vi "KEY_PRESS.vi"(0 "device ID":refnum<k1>, 1 "error in (no error)":errorcluster) -> (2 "device ID 2":refnum<k1>, 3 "Direction 2":T1, 4 "error out":errorcluster)   [LabVIEW 2015]
uses:
  DIR GAME.ctl
  <vilib>/Utility/inputDevices.llb/keyboardAcquire.vi
panel:
  out "keys pressed 2":T2(array[ring])
  out "keys pressed":T2(array[ring])
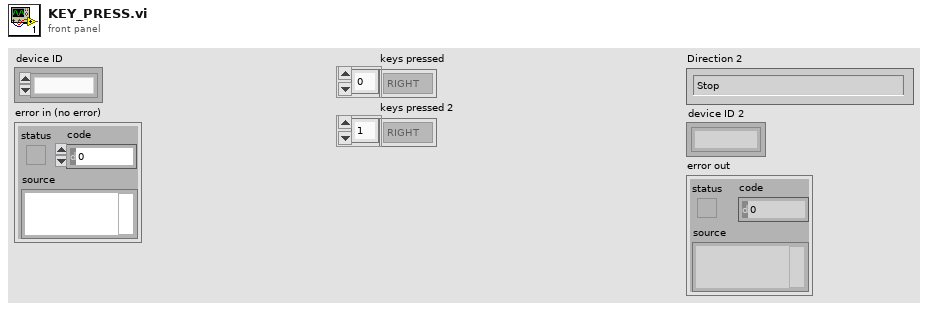
[diagram p1: front panel]
types:
  T1 = typedef "DIR GAME.ctl" = enum16{"Stop", "Front", "FR", "Right", "BR", "Back", "BL", "Left", "FL"}
  T2 = enum16{"0", "1", "2", "3", "4", "5", "6", "7", "8", "9", "A", "B", "C", "D", "E", "F", "G", "H", "I", "J", "K", "L", "M", "N", "O", "P", "Q", "R", "S", "T", "U", "V", "W", "X", "Y", "Z", "F1", "F2", "F3", "F4", "F5", "F6", "F7", "F8", "F9", "F10", "F11", "F12", "F13", "F14", "F15", "ADD", "BACK", "BACKSLASH", "CAPITAL", "COMMA", "DECIMAL", "DELETE", "DIVIDE", "DOWN", "END", "EQUALS", "ESCAPE", "GRAVE (`)", "HOME", "INSERT", "LBRACKET", "LCONTROL", "LEFT", "L ALT", "LSHIFT", "LWIN", "MINUS", "MULTIPLY", "NEXT", "NUMLOCK", "NUMPAD_0", "NUMPAD_1", "NUMPAD_2", "NUMPAD_3", "NUMPAD_4", "NUMPAD_5", "NUMPAD_6", "NUMPAD_7", "NUMPAD_8", "NUMPAD_9", "PAUSE", "PERIOD", "PRIOR (PG UP)", "RBRACKET", "RCONTROL", "RETURN", "RIGHT", "R ALT", "RSHIFT", "RWIN", "SCROLL", "SEMICOLON", "SLASH", "SPACE", "SUBTRACT", "TAB", "UP", "ENTER (num pad)", "' (quote)"}[]
  T3 = enum16{"0", "1", "2", "3", "4", "5", "6", "7", "8", "9", "A", "B", "C", "D", "E", "F", "G", "H", "I", "J", "K", "L", "M", "N", "O", "P", "Q", "R", "S", "T", "U", "V", "W", "X", "Y", "Z", "F1", "F2", "F3", "F4", "F5", "F6", "F7", "F8", "F9", "F10", "F11", "F12", "F13", "F14", "F15", "ADD", "BACK", "BACKSLASH", "CAPITAL", "COMMA", "DECIMAL", "DELETE", "DIVIDE", "DOWN", "END", "EQUALS", "ESCAPE", "GRAVE (`)", "HOME", "INSERT", "LBRACKET", "LCONTROL", "LEFT", "L ALT", "LSHIFT", "LWIN", "MINUS", "MULTIPLY", "NEXT", "NUMLOCK", "NUMPAD_0", "NUMPAD_1", "NUMPAD_2", "NUMPAD_3", "NUMPAD_4", "NUMPAD_5", "NUMPAD_6", "NUMPAD_7", "NUMPAD_8", "NUMPAD_9", "PAUSE", "PERIOD", "PRIOR (PG UP)", "RBRACKET", "RCONTROL", "RETURN", "RIGHT", "R ALT", "RSHIFT", "RWIN", "SCROLL", "SEMICOLON", "SLASH", "SPACE", "SUBTRACT", "TAB", "UP", "ENTER (num pad)", "' (quote)"}
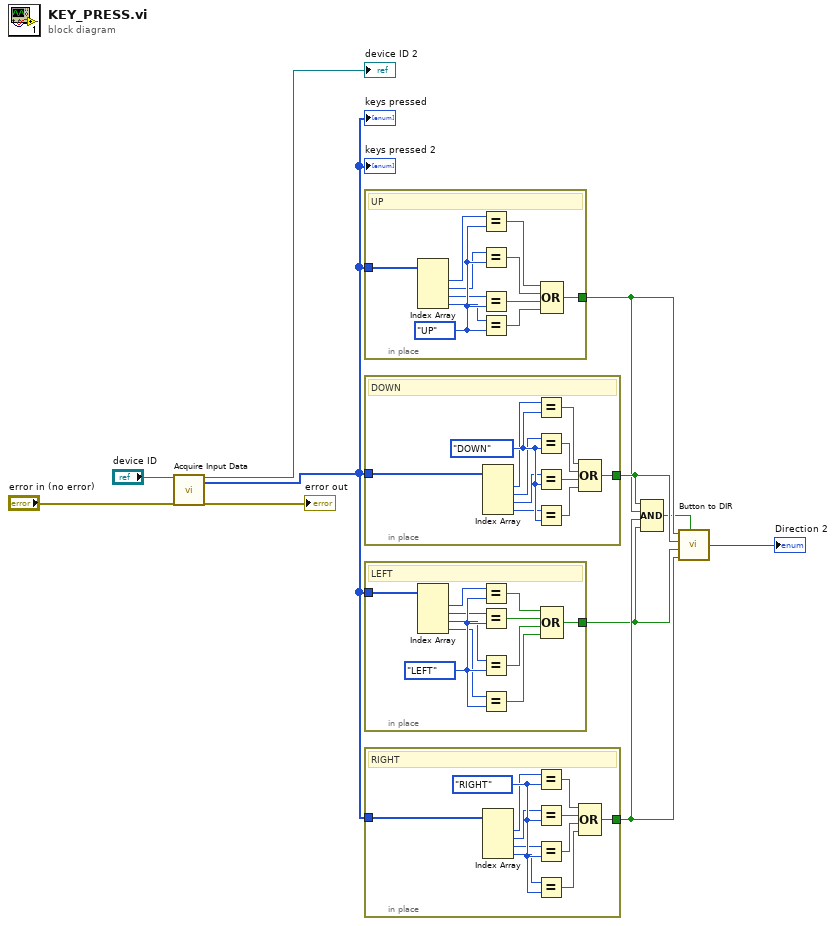
[diagram p0: block diagram]
diagram:
  n1 = call-poly <vilib>:"Acquire Input Data.vi"("device ID"="device ID", "error in (no error)"="error in (no error)") -> ("device ID"=→"device ID 2":refnum<k1>, "keys pressed"=w5:T2, "error out"=→"error out":errorcluster)  [unwired: 15 in]
  "keys pressed" <- w5
  "keys pressed 2" <- w5
  n2 = in-place {
    in-place-border: w5 -> [w13]
    in-place-border: [w12] -> w7
    w18 = T3."UP" ("element")
    # "UP"
    n3 = Index Array(array=w13) -> (element #1=w17:T3, element #2=w16:T3, element #3=w15:T3, element #4=w14:T3)  [unwired: 4 in]
    n4 = Equal?(x=w17, y=w18) -> (x = y?=w22:bool)
    n5 = Equal?(x=w16, y=w18) -> (x = y?=w21:bool)
    n6 = Equal?(x=w15, y=w18) -> (x = y?=w20:bool)
    n7 = Equal?(x=w14, y=w18) -> (x = y?=w19:bool)
    n8 = Compound Arithmetic op=OR(w22, w21, w20, w19) -> (w12:bool)
  }
  n9 = in-place {
    in-place-border: w5 -> [w24]
    in-place-border: [w23] -> w8
    w29 = T3."DOWN" ("element")
    # "DOWN"
    n10 = Index Array(array=w24) -> (element #1=w28:T3, element #2=w27:T3, element #3=w26:T3, element #4=w25:T3)  [unwired: 4 in]
    n11 = Equal?(x=w28, y=w29) -> (x = y?=w33:bool)
    n12 = Equal?(x=w27, y=w29) -> (x = y?=w32:bool)
    n13 = Equal?(x=w26, y=w29) -> (x = y?=w31:bool)
    n14 = Equal?(x=w25, y=w29) -> (x = y?=w30:bool)
    n15 = Compound Arithmetic op=OR(w33, w32, w31, w30) -> (w23:bool)
  }
  n16 = in-place {
    in-place-border: w5 -> [w35]
    in-place-border: [w34] -> w9
    w40 = T3."LEFT" ("element")
    # "LEFT"
    n17 = Index Array(array=w35) -> (element #1=w39:T3, element #2=w38:T3, element #3=w37:T3, element #4=w36:T3)  [unwired: 4 in]
    n18 = Equal?(x=w39, y=w40) -> (x = y?=w44:bool)
    n19 = Equal?(x=w38, y=w40) -> (x = y?=w43:bool)
    n20 = Equal?(x=w37, y=w40) -> (x = y?=w42:bool)
    n21 = Equal?(x=w36, y=w40) -> (x = y?=w41:bool)
    n22 = Compound Arithmetic op=OR(w44, w43, w42, w41) -> (w34:bool)
  }
  n23 = in-place {
    in-place-border: w5 -> [w46]
    in-place-border: [w45] -> w10
    w51 = T3."RIGHT" ("element")
    # "RIGHT"
    n24 = Index Array(array=w46) -> (element #1=w50:T3, element #2=w49:T3, element #3=w48:T3, element #4=w47:T3)  [unwired: 4 in]
    n25 = Equal?(x=w50, y=w51) -> (x = y?=w55:bool)
    n26 = Equal?(x=w49, y=w51) -> (x = y?=w54:bool)
    n27 = Equal?(x=w48, y=w51) -> (x = y?=w53:bool)
    n28 = Equal?(x=w47, y=w51) -> (x = y?=w52:bool)
    n29 = Compound Arithmetic op=OR(w55, w54, w53, w52) -> (w45:bool)
  }
  n30 = Compound Arithmetic op=AND(w8, w7, w10, w9) -> (w6:bool)
  n31 = call "Button to DIR.vi"("Front"=w7, "Back"=w8, "Left"=w9, "Right"=w10, "Stop Button"=w6) -> ("Direction 2"=→"Direction 2":T1)
